vi "Untitled 1.vi"() -> ()   [LabVIEW 2019]
panel:
  in  "stop":bool
  out "Numeric":dbl
  in  "Boolean":bool
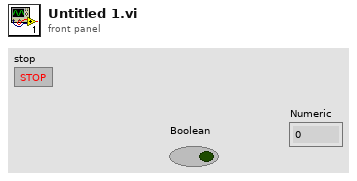
[diagram p1: front panel]
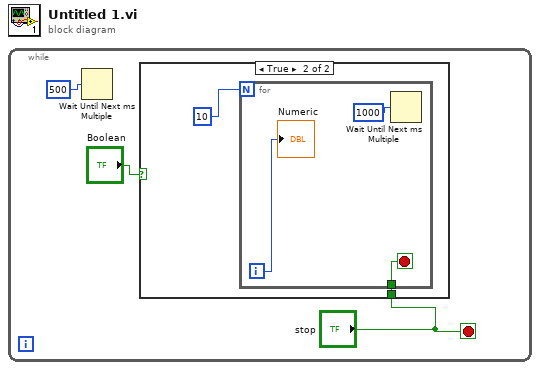
[diagram p0: block diagram]
diagram:
  n1 = while {
    stop <- "stop" stop-if-true
    n2 = Wait Until Next ms Multiple(millisecond multiple=500) -> ()  [unwired: 1 out]
    n3 = case shown="True" "Boolean" {
      tunnel: "stop" -> [_ w4]
      frame False {
      }
      frame True {
        n4 = for {
          N: 10 -> [_]
          tunnel: w4 -> [w6]
          i -> [w8]
          stop <- w6 stop-if-true
          n5 = Wait Until Next ms Multiple(millisecond multiple=1000) -> ()  [unwired: 1 out]
          "Numeric" <- w8
        }
      }
    }
  }
